vi "WPL_open waveform.vi"(5 "Command":T1, 6 "Access":T2, 7 "Variant in":variant, 8 "error in (no error)":errorcluster, 9 "dt":dbl, 10 "WFM Data Idx":i32[](array[numeric]), 11 "WPL Comm in":refnum<class "WPL Comm.lvclass">) -> (0 "error out":errorcluster, 3 "WPL Comm out":refnum<class "WPL Comm.lvclass">)   [LabVIEW 2020, in "Internal Comm Classes.lvlib" / "WPL Comm.lvclass"]
uses:
  WPL Comm.lvclass
  Access mode.ctl
  WPL Command.ctl
  WPL Comm.lvclass/WPL Comm.ctl
  Convert Q Error to Shutdown Error.vi
  <vilib>/Utility/error.llb/Error Cluster From Error Code.vi
  NI_VS Custom Device Waveform API.lvlib
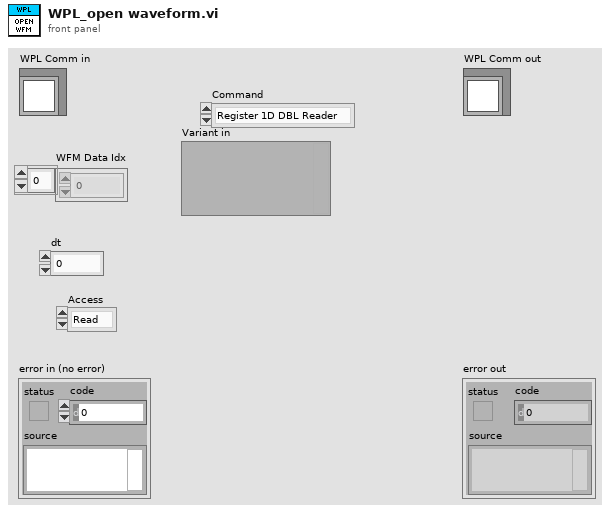
[diagram p1: front panel]
types:
  T1 = typedef "Internal Comm Classes.lvlib/WPL Comm.lvclass/WPL Command.ctl" = enum16{"Register 1D DBL Reader", "Unregister 1D DBL Reader", "Register 1D DBL Writer", "Register 2D DBL Writer", "Unregister 1D DBL Writer", "Unregister 2D DBL Writer", "DBL WFM Start", "WFM 1D DBL Data", "WFM 2D DBL Data", "Shut down", "Handle Error", "Register 1D CDB Reader", "Unregister 1D CDB Reader", "Register 1D CDB Writer", "Unregister 1D CDB Writer", "Register 2D CDB Writer", "Unregister 2D CDB Writer", "WFM 1D CDB Data", "WFM 2D CDB Data", "CDB WFM Start", "Error Shutdown", "Register Streams", "Unregister Streams", "Delete All Streams", "Get WFM DTs", "DBL WFM Multi Start", "CDB WFM Multi Start"}
  T2 = typedef "NI_VS Custom Device Waveform API.lvlib/Access mode.ctl" = enum16{"Read", "Write"}
  T3 = cluster{"Command":enum16{"Register 1D DBL Reader", "Unregister 1D DBL Reader", "Register 1D DBL Writer", "Register 2D DBL Writer", "Unregister 1D DBL Writer", "Unregister 2D DBL Writer", "DBL WFM Start", "WFM 1D DBL Data", "WFM 2D DBL Data", "Shut down", "Handle Error", "Register 1D CDB Reader", "Unregister 1D CDB Reader", "Register 1D CDB Writer", "Unregister 1D CDB Writer", "Register 2D CDB Writer", "Unregister 2D CDB Writer", "WFM 1D CDB Data", "WFM 2D CDB Data", "CDB WFM Start", "Error Shutdown", "Register Streams", "Unregister Streams", "Delete All Streams", "Get WFM DTs", "DBL WFM Multi Start", "CDB WFM Multi Start"}, "Data":variant, "Idxs":i32[], "SampleOffset":u64}
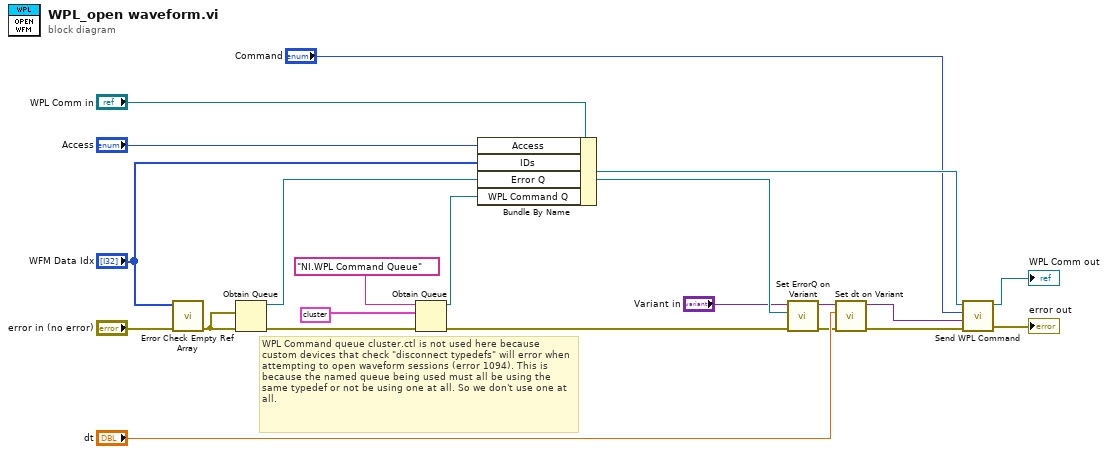
[diagram p0: block diagram]
diagram:
  # "WPL Command queue cluster.ctl is not used here because custom devices that check \"disconnect typedefs\" will error when attempting to open waveform sessions (error 1094). This is because the named queue being used must all be using the same typedef or not be using one at all. So we don't use one at all."
  n1 = call "Error Check Empty Ref Array.vi"("error in (no error)"="error in (no error)", "IDs"="WFM Data Idx") -> ("error out"=w8:errorcluster)  [unwired: 8 in, 1 out]
  n2 = Obtain Queue(element data type=w8, error in (no error)=w8) -> (queue out=w13:refnum<queue>, error out=w6:errorcluster)  [unwired: 3 in, 1 out]
  n3 = Obtain Queue(name (unnamed)="NI.WPL Command Queue", element data type=T3 {"Command"=enum."Register 1D DBL Reader", "Data"=variant, "Idxs"=[], "SampleOffset"=0} ("Queue Data"), error in (no error)=w6) -> (queue out=w14:refnum<queue>, error out=w5:errorcluster)  [unwired: 2 in, 1 out]
  n4 = Bundle By Name(cluster="WPL Comm in", "Access"="Access", "IDs"="WFM Data Idx", "Error Q"=w13, "WPL Command Q"=w14) -> (w4:refnum<class "WPL Comm.lvclass">)
  n5 = call "Set ErrorQ on Variant.vi"("error in (no error)"=w5, "Queue in"=w13, "Variant in"="Variant in") -> ("error out"=w12:errorcluster, "Variant out"=w11:variant)  [unwired: 6 in, 1 out]
  n6 = call "Set dt on Variant.vi"("error in (no error)"=w12, "dt"="dt", "Variant in"=w11) -> ("error out"=w10:errorcluster, "Variant out"=w3:variant)  [unwired: 6 in, 1 out]
  n7 = call "Send WPL Command.vi"("error in (no error)"=w10, "Variant"=w3, "Command"="Command", "WPL Comm"=w4) -> ("error out"=→"error out":errorcluster, "WPL Comm Dup"=→"WPL Comm out":refnum<class "WPL Comm.lvclass">)  [unwired: 6 in]
